vi "subSearchForAddons.vi"() -> (3 "Addons":path[](array[path]))   [LabVIEW 2020, in "DependencyInspector.lvlib" / "UIManager.lvclass"]
uses:
  UIManager.lvclass
  <vilib>/Utility/LVLibp/NI_PackedLibraryUtility.lvlib
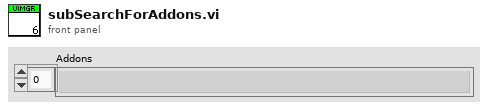
[diagram p1: front panel]
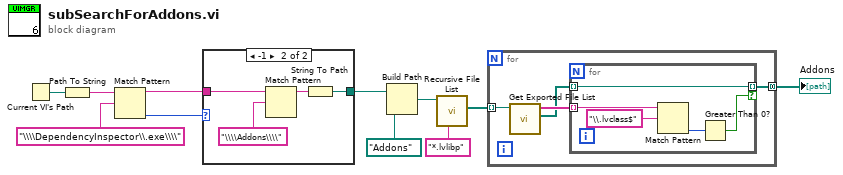
[diagram p0: block diagram]
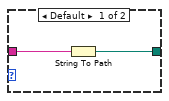
[diagram p2: hidden frame]
diagram:
  n1 = Current VI's Path() -> (path=w4:path)
  n2 = Path To String(path=w4) -> (string=w5:string)
  n3 = Match Pattern(string=w5, regular expression="\\\\DependencyInspector\\.exe\\\\") -> (before substring=w1:string, offset past match=w3:i32)  [unwired: 1 in, 2 out]
  n4 = case shown="-1" w3 {
    tunnel: w1 -> [w12 w17]
    tunnel: [w13 w14] -> w2
    frame Default {
      n5 = String To Path(string=w12) -> (path=w13:path)
    }
    frame -1 {
      n6 = Match Pattern(string=w17, regular expression="\\\\Addons\\\\") -> (before substring=w15:string)  [unwired: 1 in, 3 out]
      n7 = String To Path(string=w15) -> (path=w14:path)
    }
  }
  n8 = Build Path(base path=w2, name or relative path=path "Addons") -> (appended path=w8:path)
  n9 = call <vilib>:"Recursive File List.vi"("pattern"="*.lvlibp", "Folder Path"=w8) -> ("All Files in Dir"=w10:path[])  [unwired: 5 in, 4 out]
  n10 = for {
    tunnel: w10 -> [w21] mode=indexing
    tunnel: [w18] -> w11 mode=concatenating
    n11 = call <vilib>:"Get Exported File List.vi"("packed library path"=w21) -> ("paths"=w19:path[], "qualified names"=w20:string[])  [unwired: 8 in, 1 out]
    n12 = for {
      tunnel: w20 -> [w26] mode=indexing
      tunnel: w19 -> [w23] mode=indexing
      tunnel: [w23] -> w18 mode=indexing if=w22
      n13 = Match Pattern(string=w26, regular expression="\\.lvclass$") -> (offset past match=w24:i32)  [unwired: 1 in, 3 out]
      n14 = Greater Than 0?(x=w24) -> (x > 0?=w22:bool)
    }
  }
  "Addons" <- w11
